vi "Drivetrain Control.vi"(0 "Back Left DevRef In":T1={"DeviceStatus"={"status"=FALSE, "code"=0, "source"=""}, "Type"=enum."PWM", "PWM"={"Digital Module"=enum."Digital Module 1", "PWM Channel"=enum."Invalid", "DeadBand"={"Name"="", "maxPositivePwm"=0, "minPositivePwm"=0, "centerPwm"=0, "maxNegativePwm"=0, "minNegativePwm"=0, "angularRange"=0}}, "CAN"={"Device Number"=0, "Control Mode"=enum."Percent VBus", "Semaphore"=refnum, "Max Vout"=12.0}, "Invert"=FALSE, "TransformRef"=refnum, "InvTransformRef"=refnum}, 1 "X Axis":dbl, 2 "Y Axis":dbl, 5 "Back Right DevRef In":T1={"DeviceStatus"={"status"=FALSE, "code"=0, "source"=""}, "Type"=enum."PWM", "PWM"={"Digital Module"=enum."Digital Module 1", "PWM Channel"=enum."Invalid", "DeadBand"={"Name"="", "maxPositivePwm"=0, "minPositivePwm"=0, "centerPwm"=0, "maxNegativePwm"=0, "minNegativePwm"=0, "angularRange"=0}}, "CAN"={"Device Number"=0, "Control Mode"=enum."Percent VBus", "Semaphore"=refnum, "Max Vout"=12.0}, "Invert"=FALSE, "TransformRef"=refnum, "InvTransformRef"=refnum}, 7 "Front Left DevRef In":T1={"DeviceStatus"={"status"=FALSE, "code"=0, "source"=""}, "Type"=enum."PWM", "PWM"={"Digital Module"=enum."Digital Module 1", "PWM Channel"=enum."Invalid", "DeadBand"={"Name"="", "maxPositivePwm"=0, "minPositivePwm"=0, "centerPwm"=0, "maxNegativePwm"=0, "minNegativePwm"=0, "angularRange"=0}}, "CAN"={"Device Number"=0, "Control Mode"=enum."Percent VBus", "Semaphore"=refnum, "Max Vout"=12.0}, "Invert"=FALSE, "TransformRef"=refnum, "InvTransformRef"=refnum}, 9 "Front Right DevRef In":T1={"DeviceStatus"={"status"=FALSE, "code"=0, "source"=""}, "Type"=enum."PWM", "PWM"={"Digital Module"=enum."Digital Module 1", "PWM Channel"=enum."Invalid", "DeadBand"={"Name"="", "maxPositivePwm"=0, "minPositivePwm"=0, "centerPwm"=0, "maxNegativePwm"=0, "minNegativePwm"=0, "angularRange"=0}}, "CAN"={"Device Number"=0, "Control Mode"=enum."Percent VBus", "Semaphore"=refnum, "Max Vout"=12.0}, "Invert"=FALSE, "TransformRef"=refnum, "InvTransformRef"=refnum}, 11 "Closed Loop On/Off":bool, 12 "Drivetrain Reverse Button":bool, 13 "Aim To Target":bool) -> (3 "Left Motor Value":dbl, 4 "Back Left DevRef Out":T1={"DeviceStatus"={"status"=FALSE, "code"=0, "source"=""}, "Type"=enum."PWM", "PWM"={"Digital Module"=enum."Digital Module 1", "PWM Channel"=enum."Invalid", "DeadBand"={"Name"="", "maxPositivePwm"=0, "minPositivePwm"=0, "centerPwm"=0, "maxNegativePwm"=0, "minNegativePwm"=0, "angularRange"=0}}, "CAN"={"Device Number"=0, "Control Mode"=enum."Percent VBus", "Semaphore"=refnum, "Max Vout"=12.0}, "Invert"=FALSE, "TransformRef"=refnum, "InvTransformRef"=refnum}, 6 "Back Right DevRef Out":T1={"DeviceStatus"={"status"=FALSE, "code"=0, "source"=""}, "Type"=enum."PWM", "PWM"={"Digital Module"=enum."Digital Module 1", "PWM Channel"=enum."Invalid", "DeadBand"={"Name"="", "maxPositivePwm"=0, "minPositivePwm"=0, "centerPwm"=0, "maxNegativePwm"=0, "minNegativePwm"=0, "angularRange"=0}}, "CAN"={"Device Number"=0, "Control Mode"=enum."Percent VBus", "Semaphore"=refnum, "Max Vout"=12.0}, "Invert"=FALSE, "TransformRef"=refnum, "InvTransformRef"=refnum}, 8 "Front Left DevRef Out":T1={"DeviceStatus"={"status"=FALSE, "code"=0, "source"=""}, "Type"=enum."PWM", "PWM"={"Digital Module"=enum."Digital Module 1", "PWM Channel"=enum."Invalid", "DeadBand"={"Name"="", "maxPositivePwm"=0, "minPositivePwm"=0, "centerPwm"=0, "maxNegativePwm"=0, "minNegativePwm"=0, "angularRange"=0}}, "CAN"={"Device Number"=0, "Control Mode"=enum."Percent VBus", "Semaphore"=refnum, "Max Vout"=12.0}, "Invert"=FALSE, "TransformRef"=refnum, "InvTransformRef"=refnum}, 10 "Front Right DevRef Out":T1={"DeviceStatus"={"status"=FALSE, "code"=0, "source"=""}, "Type"=enum."PWM", "PWM"={"Digital Module"=enum."Digital Module 1", "PWM Channel"=enum."Invalid", "DeadBand"={"Name"="", "maxPositivePwm"=0, "minPositivePwm"=0, "centerPwm"=0, "maxNegativePwm"=0, "minNegativePwm"=0, "angularRange"=0}}, "CAN"={"Device Number"=0, "Control Mode"=enum."Percent VBus", "Semaphore"=refnum, "Max Vout"=12.0}, "Invert"=FALSE, "TransformRef"=refnum, "InvTransformRef"=refnum}, 14 "Right Motor Value":dbl)   [LabVIEW 2012]
uses:
  <vilib>/Rock Robotics/WPI/MotorControl/WPI_MotorControlDeviceRef.ctl
  <vilib>/Rock Robotics/SystemInterfaces/Typedef/FPGA_TypedefDigitalModule.ctl
  <vilib>/Rock Robotics/SystemInterfaces/DIO/FPGA_DIOPWMChannel.ctl
  <vilib>/Rock Robotics/WPI/PWM/WPI_PWMDeadband.ctl
  <vilib>/Rock Robotics/WPI/CAN/Jaguar/SubVIs/WPI_CANJaguar_ControlMode.ctl
  <vilib>/Rock Robotics/WPI/PWM/WPI_PWMTransform_ConPane.ctl
  <vilib>/Rock Robotics/WPI/DriverStation/DriverStationLCD/WPI_DriverStationLCDLCDLine.ctl
  <vilib>/Rock Robotics/WPI/CAN/Jaguar/SubVIs/WPI_CANJaguar_SpeedReference.ctl
  Robot Global Data.vi
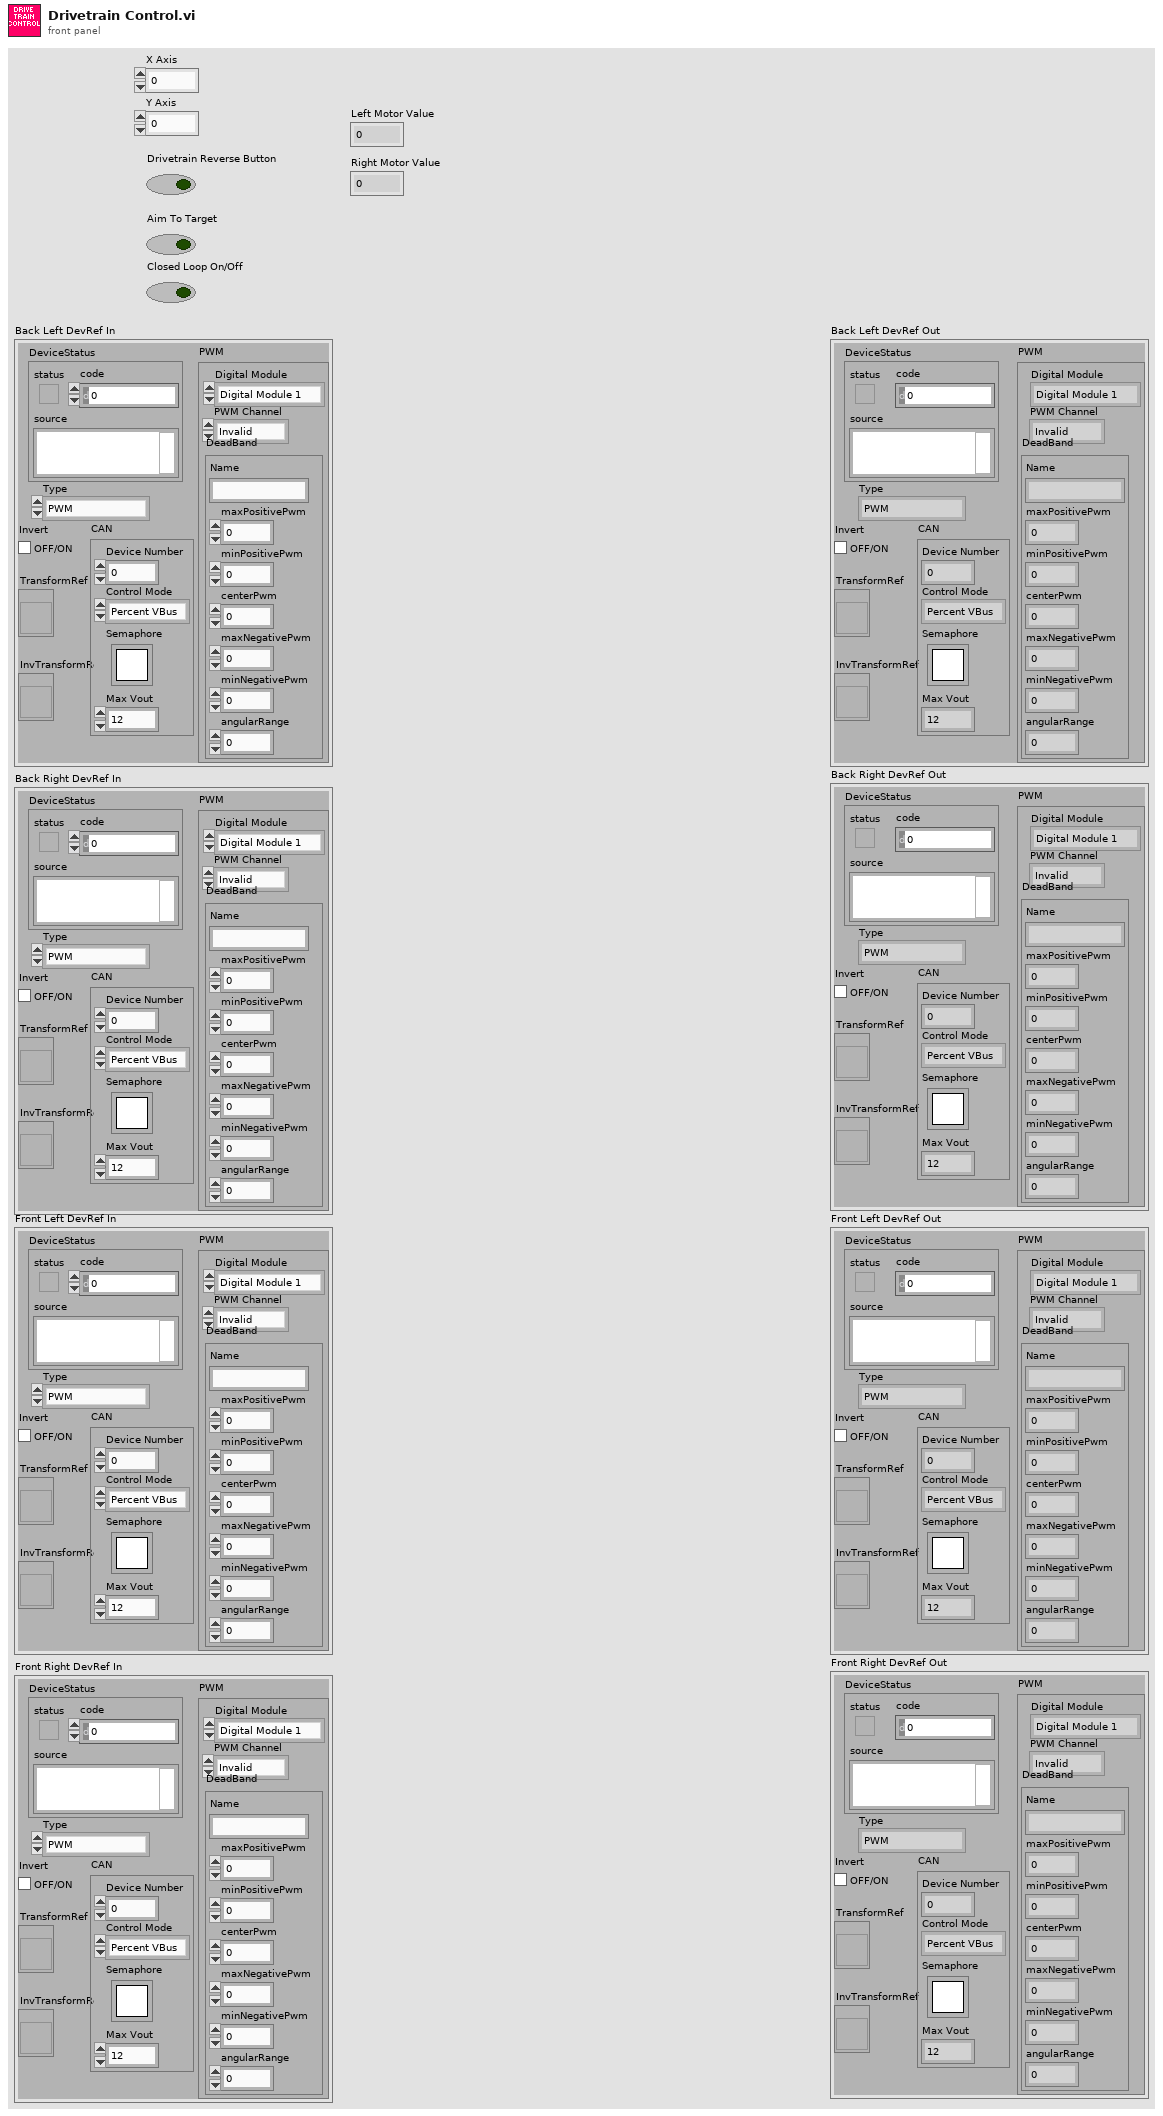
[diagram p1: front panel]
types:
  T1 = typedef "WPI_MotorControlDeviceRef.ctl" = cluster{"DeviceStatus":errorcluster, "Type":enum16{"PWM", "CAN"}, "PWM":cluster{"Digital Module":T2, "PWM Channel":T3, "DeadBand":T4}, "CAN":cluster{"Device Number":u8, "Control Mode":T5, "Semaphore":T6, "Max Vout":dbl}, "Invert":bool, "TransformRef":T7, "InvTransformRef":T7}
  T2 = typedef "FPGA_TypedefDigitalModule.ctl" = enum16{"Digital Module 1", "Digital Module 2"}
  T3 = typedef "FPGA_DIOPWMChannel.ctl" = enum8{"PWM 1", "PWM 2", "PWM 3", "PWM 4", "PWM 5", "PWM 6", "PWM 7", "PWM 8", "PWM 9", "PWM 10", "Invalid"}
  T4 = typedef "WPI_PWMDeadband.ctl" = cluster{"Name":string, "maxPositivePwm":i32, "minPositivePwm":i32, "centerPwm":i32, "maxNegativePwm":i32, "minNegativePwm":i32, "angularRange":u16}
  T5 = typedef "WPI_CANJaguar_ControlMode.ctl" = enum8{"Percent VBus", "Current", "Speed", "Position", "Voltage"}
  T6 = typedef "Semaphore RefNum" = refnum<k1>
  T7 = typedef "WPI_PWMTransform_ConPane.ctl" = refnum<vi>
  T8 = typedef "WPI_DriverStationLCDLCDLine.ctl" = enum16{"Main - Line 1", "User - Line 2", "User - Line 3", "User - Line 4", "User - Line 5", "User - Line 6"}
  T9 = typedef "WPI_CANJaguar_SpeedReference.ctl" = u8
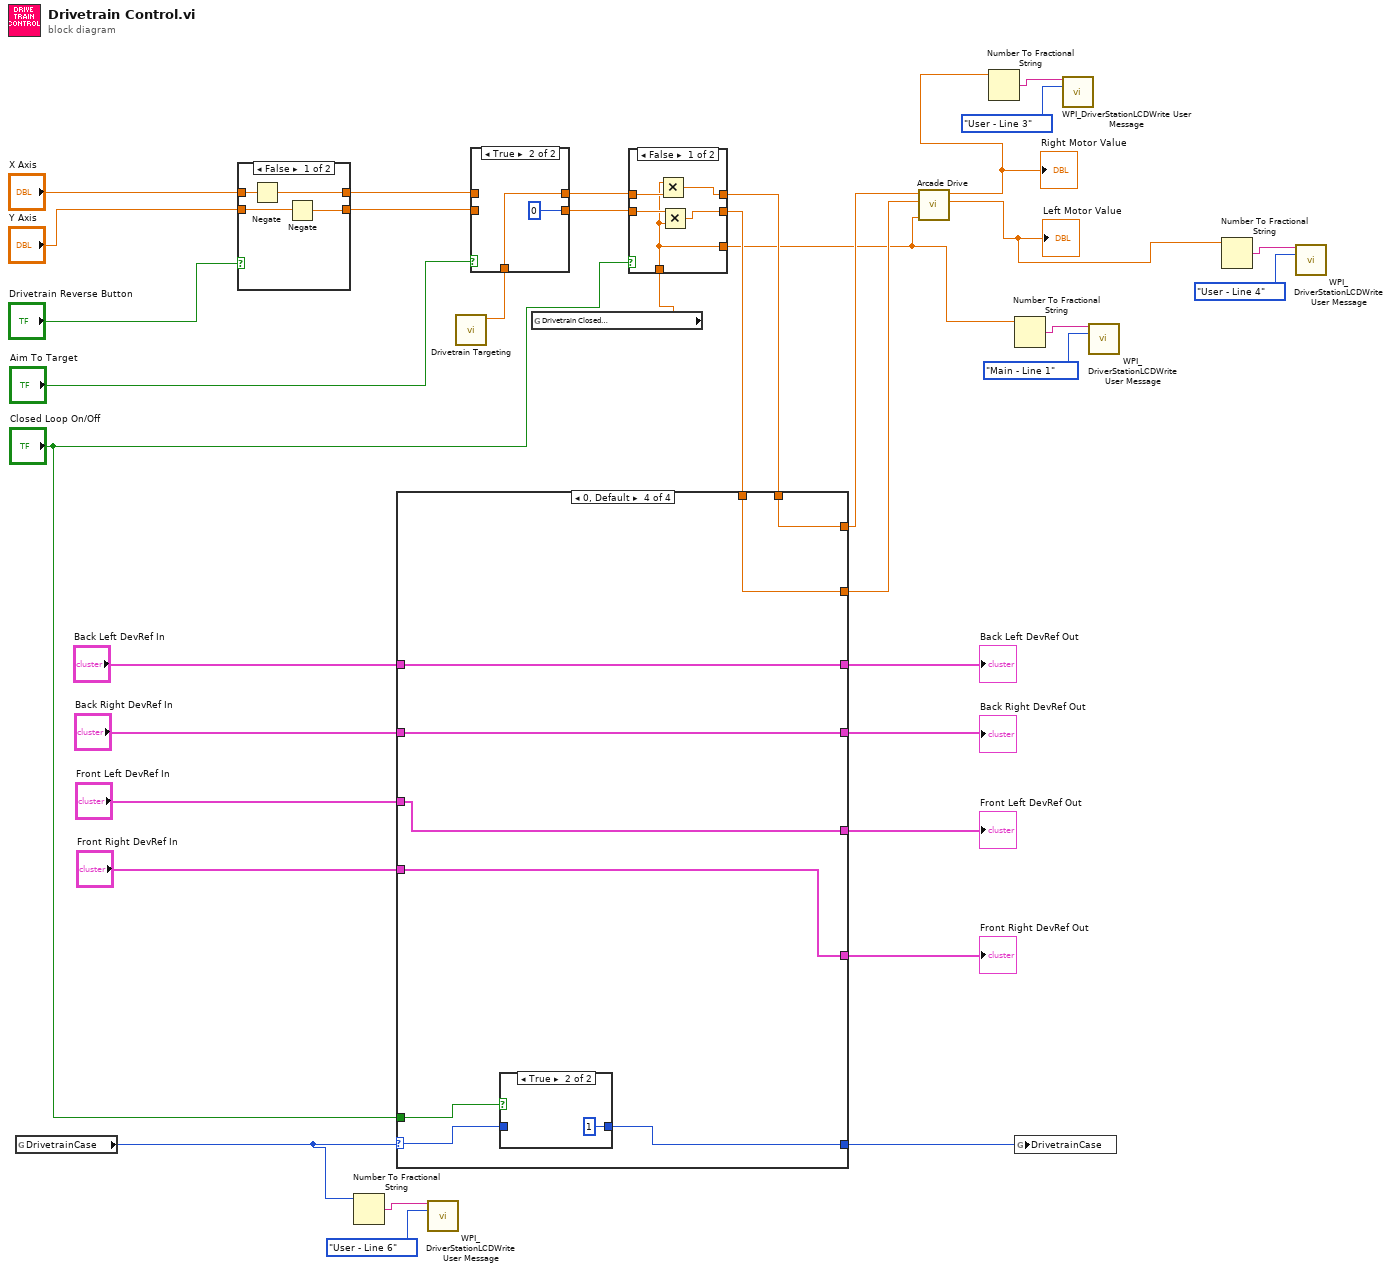
[diagram p0: block diagram]
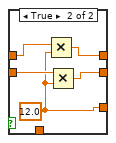
[diagram p2: hidden frame]
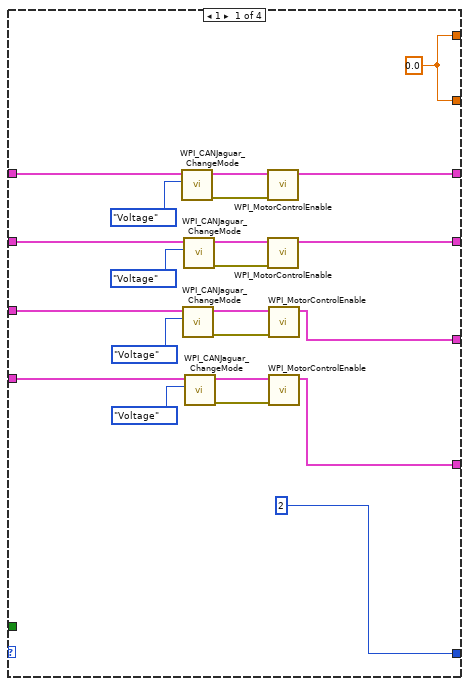
[diagram p3: hidden frame]
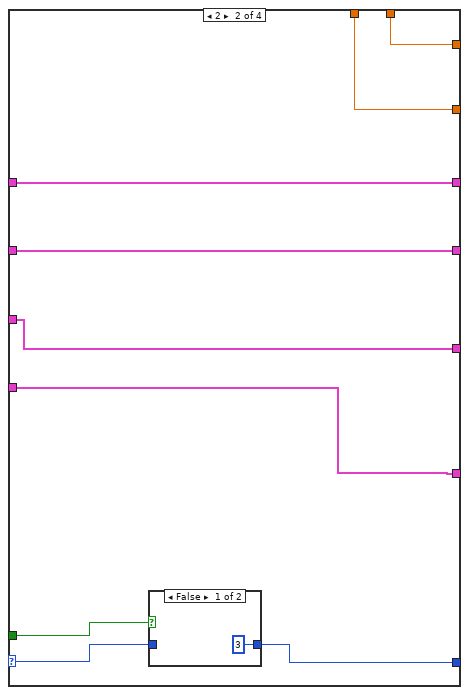
[diagram p4: hidden frame]
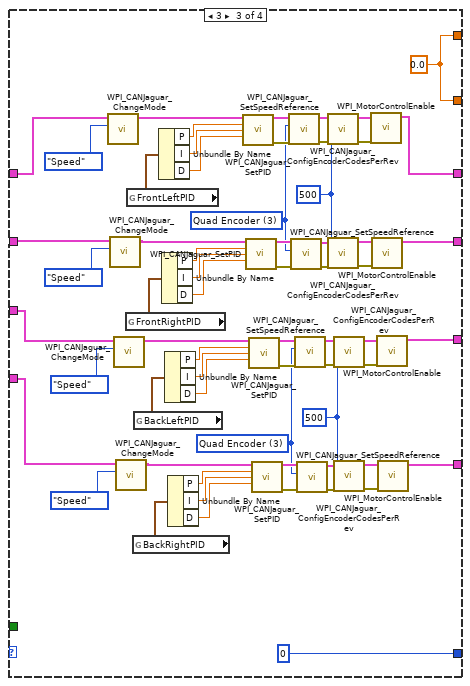
[diagram p6: hidden frame]
diagram:
  n1 = global read "Robot Global Data.vi" "DrivetrainCase"() -> (w1:i8)
  n2 = case shown="False" "Drivetrain Reverse Button" {
    tunnel: [w37 w42] -> w36
    tunnel: "X Axis" -> [w40 w42]
    tunnel: [w38 w41] -> w35
    tunnel: "Y Axis" -> [w39 w41]
    frame False {
      n3 = Negate(x=w40) -> (-x=w37:dbl)
      n4 = Negate(x=w39) -> (-x=w38:dbl)
    }
    frame True {
    }
  }
  n5 = Number To Fractional String(number=w1) -> (F-format string=w3:string)  [unwired: 3 in]
  n6 = call <vilib>:"WPI_DriverStationLCDWrite User Message.vi"("line text"=w3, "line"=WPI_DriverStationLCDLCDLine."User - Line 6") -> ()  [unwired: 13 in, 1 out]
  n7 = call "Drivetrain Targeting.vi"() -> ("X Axis Out"=w31:dbl)  [unwired: 11 in]
  n8 = case shown="True" "Aim To Target" {
    tunnel: [w44 w45] -> w29
    tunnel: w36 -> [w44 _]
    tunnel: [w43 0] -> w28
    tunnel: w35 -> [w43 _]
    tunnel: w31 -> [_ w45]
    frame False {
    }
    frame True {
    }
  }
  n9 = global read "Robot Global Data.vi" "Drivetrain Closed\nLoop Max"() -> (w27:dbl)
  n10 = case shown="False" "Closed Loop On/Off" {
    tunnel: [w49 w54] -> w25
    tunnel: w29 -> [w51 w56]
    tunnel: [w48 w53] -> w26
    tunnel: w28 -> [w50 w55]
    tunnel: w27 -> [w47 _]
    tunnel: [w47 w52] -> w10
    frame False {
      n11 = Multiply(x=w47, y=w51) -> (x*y=w49:dbl)
      n12 = Multiply(x=w50, y=w47) -> (x*y=w48:dbl)
    }
    frame True {
      w52 = 12.0
      n13 = Multiply(x=w56, y=w52) -> (x*y=w54:dbl)
      n14 = Multiply(x=w55, y=w52) -> (x*y=w53:dbl)
    }
  }
  n15 = case shown="0, Default" w1 {
    selector: w1 -> [_ w84 _ w156]
    tunnel: [i8 2 ("ShooterCase") w83 i8 0 ("ShooterCase") w157] -> w30
    tunnel: "Back Left DevRef In" -> [w77 w87 w149 w160]
    tunnel: "Back Right DevRef In" -> [w76 w86 w148 w159]
    tunnel: [w69 w87 w121 w160] -> w17
    tunnel: [w68 w86 w122 w159] -> w16
    tunnel: "Closed Loop On/Off" -> [_ w85 _ w158]
    tunnel: w25 -> [_ w81 _ w155]
    tunnel: w26 -> [_ w82 _ w154]
    tunnel: [w67 w81 w120 w155] -> w24
    tunnel: [w67 w82 w120 w154] -> w23
    tunnel: "Front Left DevRef In" -> [w60 w80 w93 w153]
    tunnel: "Front Right DevRef In" -> [w59 w79 w92 w152]
    tunnel: [w58 w80 w91 w153] -> w15
    tunnel: [w57 w79 w90 w152] -> w14
    frame 1 {
      w67 = 0.0 ("FSpeed")
      n16 = call <vilib>:"WPI_CANJaguar_ChangeMode.vi"("Control Mode"=WPI_CANJaguar_ControlMode."Voltage", "CAN Jaguar Ref"=w77) -> ("error out"=w70:errorcluster, "CAN Jaguar Ref Out"=w71:T1)  [unwired: 8 in]
      n17 = call <vilib>:"WPI_CANJaguar_ChangeMode.vi"("Control Mode"=WPI_CANJaguar_ControlMode."Voltage", "CAN Jaguar Ref"=w60) -> ("error out"=w61:errorcluster, "CAN Jaguar Ref Out"=w62:T1)  [unwired: 8 in]
      n18 = call <vilib>:"WPI_CANJaguar_ChangeMode.vi"("Control Mode"=WPI_CANJaguar_ControlMode."Voltage", "CAN Jaguar Ref"=w76) -> ("error out"=w72:errorcluster, "CAN Jaguar Ref Out"=w73:T1)  [unwired: 8 in]
      n19 = call <vilib>:"WPI_CANJaguar_ChangeMode.vi"("Control Mode"=WPI_CANJaguar_ControlMode."Voltage", "CAN Jaguar Ref"=w59) -> ("error out"=w63:errorcluster, "CAN Jaguar Ref Out"=w64:T1)  [unwired: 8 in]
      n20 = call <vilib>:"WPI_MotorControlEnable.vi"("error in (no error)"=w70, "CAN Jaguar Ref"=w71) -> ("CAN Jaguar Ref Out"=w69:T1)  [unwired: 8 in, 1 out]
      n21 = call <vilib>:"WPI_MotorControlEnable.vi"("error in (no error)"=w72, "CAN Jaguar Ref"=w73) -> ("CAN Jaguar Ref Out"=w68:T1)  [unwired: 8 in, 1 out]
      n22 = call <vilib>:"WPI_MotorControlEnable.vi"("error in (no error)"=w61, "CAN Jaguar Ref"=w62) -> ("CAN Jaguar Ref Out"=w58:T1)  [unwired: 8 in, 1 out]
      n23 = call <vilib>:"WPI_MotorControlEnable.vi"("error in (no error)"=w63, "CAN Jaguar Ref"=w64) -> ("CAN Jaguar Ref Out"=w57:T1)  [unwired: 8 in, 1 out]
    }
    frame 2 {
      n24 = case shown="False" w85 {
        tunnel: [i8 3 ("ShooterCase") w89] -> w83
        tunnel: w84 -> [_ w89]
        frame False {
        }
        frame True {
        }
      }
    }
    frame 3 {
      w98 = u16 500 ("Encoder Codes Per Rev")
      w103 = T9 3 items=["Encoder"=0, "Inv Encoder"=2, "Quad Encoder"=3, "None"=255] ("Speed Reference")
      w120 = 0.0 ("FSpeed")
      w127 = u16 500 ("Encoder Codes Per Rev")
      w132 = T9 3 items=["Encoder"=0, "Inv Encoder"=2, "Quad Encoder"=3, "None"=255] ("Speed Reference")
      n25 = call <vilib>:"WPI_CANJaguar_ChangeMode.vi"("Control Mode"=WPI_CANJaguar_ControlMode."Speed", "CAN Jaguar Ref"=w149) -> ("CAN Jaguar Ref Out"=w147:T1)  [unwired: 8 in, 1 out]
      n26 = call <vilib>:"WPI_CANJaguar_ChangeMode.vi"("Control Mode"=WPI_CANJaguar_ControlMode."Speed", "CAN Jaguar Ref"=w148) -> ("CAN Jaguar Ref Out"=w138:T1)  [unwired: 8 in, 1 out]
      n27 = call <vilib>:"WPI_CANJaguar_ChangeMode.vi"("Control Mode"=WPI_CANJaguar_ControlMode."Speed", "CAN Jaguar Ref"=w93) -> ("CAN Jaguar Ref Out"=w117:T1)  [unwired: 8 in, 1 out]
      n28 = call <vilib>:"WPI_CANJaguar_ChangeMode.vi"("Control Mode"=WPI_CANJaguar_ControlMode."Speed", "CAN Jaguar Ref"=w92) -> ("CAN Jaguar Ref Out"=w108:T1)  [unwired: 8 in, 1 out]
      n29 = global read "Robot Global Data.vi" "FrontRightPID"() -> (w142:cluster{"P":dbl, "I":dbl, "D":dbl})
      n30 = global read "Robot Global Data.vi" "FrontLeftPID"() -> (w146:cluster{"P":dbl, "I":dbl, "D":dbl})
      n31 = global read "Robot Global Data.vi" "BackRightPID"() -> (w112:cluster{"P":dbl, "I":dbl, "D":dbl})
      n32 = global read "Robot Global Data.vi" "BackLeftPID"() -> (w116:cluster{"P":dbl, "I":dbl, "D":dbl})
      n33 = Unbundle By Name(w146) -> ("P"=w145:dbl, "I"=w144:dbl, "D"=w143:dbl)
      n34 = Unbundle By Name(w142) -> ("P"=w141:dbl, "I"=w140:dbl, "D"=w139:dbl)
      n35 = Unbundle By Name(w116) -> ("P"=w115:dbl, "I"=w114:dbl, "D"=w113:dbl)
      n36 = Unbundle By Name(w112) -> ("P"=w111:dbl, "I"=w110:dbl, "D"=w109:dbl)
      n37 = call <vilib>:"WPI_CANJaguar_SetPID.vi"("CAN Jaguar Ref"=w147, "P"=w145, "I"=w144, "D"=w143) -> ("CAN Jaguar Ref Out"=w135:T1, "error out"=w136:errorcluster)  [unwired: 10 in]
      n38 = call <vilib>:"WPI_CANJaguar_SetPID.vi"("CAN Jaguar Ref"=w138, "P"=w141, "I"=w140, "D"=w139) -> ("CAN Jaguar Ref Out"=w134:T1, "error out"=w133:errorcluster)  [unwired: 10 in]
      n39 = call <vilib>:"WPI_CANJaguar_SetPID.vi"("CAN Jaguar Ref"=w117, "P"=w115, "I"=w114, "D"=w113) -> ("CAN Jaguar Ref Out"=w106:T1, "error out"=w107:errorcluster)  [unwired: 10 in]
      n40 = call <vilib>:"WPI_CANJaguar_SetPID.vi"("CAN Jaguar Ref"=w108, "P"=w111, "I"=w110, "D"=w109) -> ("CAN Jaguar Ref Out"=w105:T1, "error out"=w104:errorcluster)  [unwired: 10 in]
      n41 = call <vilib>:"WPI_CANJaguar_SetSpeedReference.vi"("error in (no error)"=w136, "Speed Reference"=w132, "CAN Jaguar Ref"=w135) -> ("error out"=w131:errorcluster, "CAN Jaguar Ref Out"=w130:T1)  [unwired: 7 in]
      n42 = call <vilib>:"WPI_CANJaguar_SetSpeedReference.vi"("error in (no error)"=w133, "Speed Reference"=w132, "CAN Jaguar Ref"=w134) -> ("error out"=w128:errorcluster, "CAN Jaguar Ref Out"=w129:T1)  [unwired: 7 in]
      n43 = call <vilib>:"WPI_CANJaguar_SetSpeedReference.vi"("error in (no error)"=w107, "Speed Reference"=w103, "CAN Jaguar Ref"=w106) -> ("error out"=w102:errorcluster, "CAN Jaguar Ref Out"=w101:T1)  [unwired: 7 in]
      n44 = call <vilib>:"WPI_CANJaguar_SetSpeedReference.vi"("error in (no error)"=w104, "Speed Reference"=w103, "CAN Jaguar Ref"=w105) -> ("error out"=w99:errorcluster, "CAN Jaguar Ref Out"=w100:T1)  [unwired: 7 in]
      n45 = call <vilib>:"WPI_CANJaguar_ConfigEncoderCodesPerRev.vi"("error in (no error)"=w131, "Encoder Codes Per Rev"=w127, "CAN Jaguar Ref"=w130) -> ("error out"=w126:errorcluster, "CAN Jaguar Ref Out"=w125:T1)  [unwired: 7 in]
      n46 = call <vilib>:"WPI_CANJaguar_ConfigEncoderCodesPerRev.vi"("error in (no error)"=w128, "Encoder Codes Per Rev"=w127, "CAN Jaguar Ref"=w129) -> ("error out"=w124:errorcluster, "CAN Jaguar Ref Out"=w123:T1)  [unwired: 7 in]
      n47 = call <vilib>:"WPI_CANJaguar_ConfigEncoderCodesPerRev.vi"("error in (no error)"=w102, "Encoder Codes Per Rev"=w98, "CAN Jaguar Ref"=w101) -> ("error out"=w97:errorcluster, "CAN Jaguar Ref Out"=w96:T1)  [unwired: 7 in]
      n48 = call <vilib>:"WPI_CANJaguar_ConfigEncoderCodesPerRev.vi"("error in (no error)"=w99, "Encoder Codes Per Rev"=w98, "CAN Jaguar Ref"=w100) -> ("error out"=w95:errorcluster, "CAN Jaguar Ref Out"=w94:T1)  [unwired: 7 in]
      n49 = call <vilib>:"WPI_MotorControlEnable.vi"("error in (no error)"=w126, "CAN Jaguar Ref"=w125) -> ("CAN Jaguar Ref Out"=w121:T1)  [unwired: 8 in, 1 out]
      n50 = call <vilib>:"WPI_MotorControlEnable.vi"("error in (no error)"=w124, "CAN Jaguar Ref"=w123) -> ("CAN Jaguar Ref Out"=w122:T1)  [unwired: 8 in, 1 out]
      n51 = call <vilib>:"WPI_MotorControlEnable.vi"("error in (no error)"=w97, "CAN Jaguar Ref"=w96) -> ("CAN Jaguar Ref Out"=w91:T1)  [unwired: 8 in, 1 out]
      n52 = call <vilib>:"WPI_MotorControlEnable.vi"("error in (no error)"=w95, "CAN Jaguar Ref"=w94) -> ("CAN Jaguar Ref Out"=w90:T1)  [unwired: 8 in, 1 out]
    }
    frame 0, Default {
      n53 = case shown="True" w158 {
        tunnel: [w161 i8 1 ("ShooterCase")] -> w157
        tunnel: w156 -> [w161 _]
        frame False {
        }
        frame True {
        }
      }
    }
  }
  "Back Left DevRef Out" <- w17
  "Back Right DevRef Out" <- w16
  "Front Left DevRef Out" <- w15
  "Front Right DevRef Out" <- w14
  n54 = call "Arcade Drive.vi"("Max Output"=w10, "Y Axis"=w23, "X Axis"=w24) -> ("Left Motor Value"=w4:dbl, "Right Motor Value"=w5:dbl)  [unwired: 7 in]
  "Right Motor Value" <- w5
  "Left Motor Value" <- w4
  n55 = Number To Fractional String(number=w5) -> (F-format string=w9:string)  [unwired: 3 in]
  n56 = Number To Fractional String(number=w10) -> (F-format string=w12:string)  [unwired: 3 in]
  n57 = global write "Robot Global Data.vi" "DrivetrainCase"(w30) -> ()
  n58 = call <vilib>:"WPI_DriverStationLCDWrite User Message.vi"("line text"=w9, "line"=WPI_DriverStationLCDLCDLine."User - Line 3") -> ()  [unwired: 13 in, 1 out]
  n59 = call <vilib>:"WPI_DriverStationLCDWrite User Message.vi"("line text"=w12, "line"=WPI_DriverStationLCDLCDLine."Main - Line 1") -> ()  [unwired: 13 in, 1 out]
  n60 = Number To Fractional String(number=w4) -> (F-format string=w7:string)  [unwired: 3 in]
  n61 = call <vilib>:"WPI_DriverStationLCDWrite User Message.vi"("line text"=w7, "line"=WPI_DriverStationLCDLCDLine."User - Line 4") -> ()  [unwired: 13 in, 1 out]
